vi "Configure Dialog.vi"(8 "error in (no error)":errorcluster, 11 "Configure Standard Waveform [STD] Msg in":refnum<class "Configure Standard Waveform [STD] Msg.lvclass">) -> (0 "error out":errorcluster, 2 "Ok?":bool, 3 "Configure Standard Waveform [STD] Msg out":refnum<class "Configure Standard Waveform [STD] Msg.lvclass">)   [LabVIEW 2014, in "CS++Fgen.lvlib" / "Configure Standard Waveform [STD] Msg.lvclass"]
uses:
  Configure Standard Waveform [STD] Msg.lvclass
  Configure Standard Waveform [STD] Msg.lvclass/Configure Standard Waveform [STD] Msg.ctl
panel:
  in  "waveform (Sine)":i32(ring)=1 caption="Waveform" items=["Sine"=1, "Square"=2, "Triangle"=3, "Ramp Up"=4, "Ramp Down"=5, "DC"=6]
  in  "amplitude (1.00 V)":dbl[unit]=1.0 caption="Amplitude" format="%.3f"
  in  "channel name (\"CHANNEL1\")":string="CHANNEL1" caption="Channel Name"
  in  "dc offset (0.00 V)":dbl[unit] caption="DC Offset" format="%.3f"
  in  "frequency (1000.0 Hz)":dbl[unit]=1000.0 caption="Frequency" format="%^.2e"
  in  "start phase (0.00 Degrees)":dbl[unit] caption="Start Phase" format="%.3f"
  in  "OK Button":bool
  in  "Cancel Button":bool
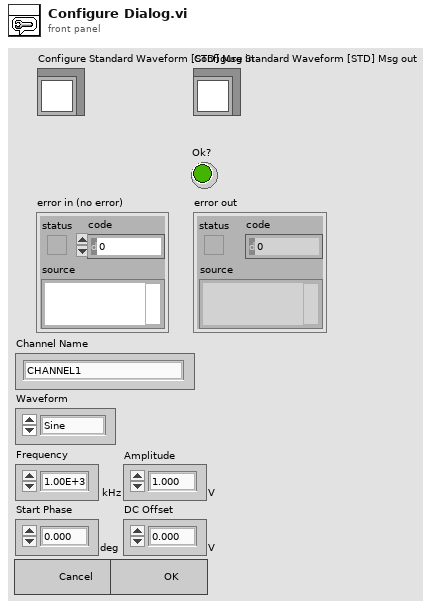
[diagram p1: front panel]
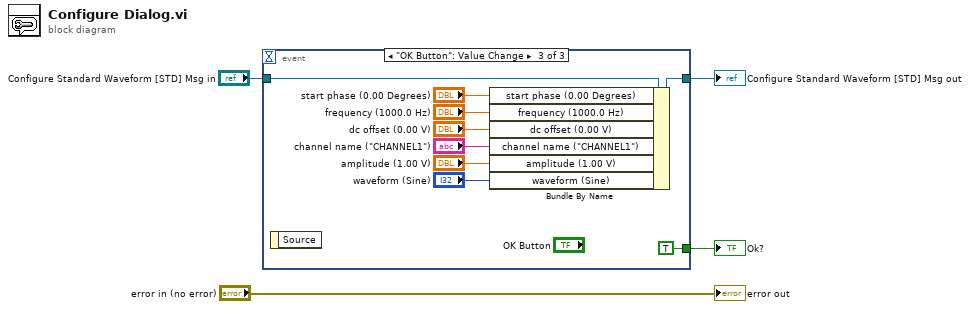
[diagram p0: block diagram]
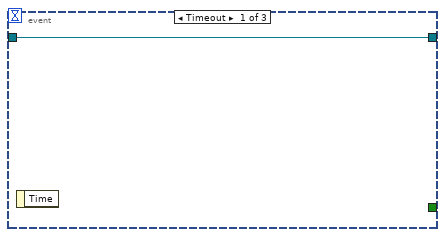
[diagram p2: hidden frame]
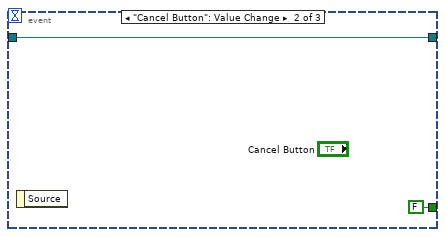
[diagram p3: hidden frame]
diagram:
  n1 = event shown="[2] \"OK Button\": Value Change" {
    selector: _ -> [_ _ _]
    dyn-events: _ -> [_ _ _]
    timeout: _ -> [_ _ _]
    tunnel: [w5 w7 w14] -> w3
    tunnel: "Configure Standard Waveform [STD] Msg in" -> [w5 w7 w15]
    tunnel: [_ FALSE TRUE] -> w1
    event Timeout {
      n2 = event-data() -> ()  [unwired: 1 in, 1 out]
    }
    event "Cancel Button": Value Change {
      n3 = event-data() -> ()  [unwired: 1 in, 1 out]
    }
    event "OK Button": Value Change {
      n4 = event-data() -> ()  [unwired: 1 in, 1 out]
      n5 = Bundle By Name(cluster=w15, "start phase (0.00 Degrees)"="start phase (0.00 Degrees)", "frequency (1000.0 Hz)"="frequency (1000.0 Hz)", "dc offset (0.00 V)"="dc offset (0.00 V)", "channel name (\"CHANNEL1\")"="channel name (\"CHANNEL1\")", "amplitude (1.00 V)"="amplitude (1.00 V)", "waveform (Sine)"="waveform (Sine)") -> (w14:refnum<class "Configure Standard Waveform [STD] Msg.lvclass">)
    }
  }
  "Configure Standard Waveform [STD] Msg out" <- w3
  "Ok?" <- w1
  "error out" <- "error in (no error)"
